vi "Field Types.vi"() -> (3 "Creatable Field Types":refnum<class "Type.lvclass">[](array[class]))   [LabVIEW 2020, in "Conditum-Tools.lvlib"]
uses:
  Conditum-Tools.lvlib
  Conditum-Clone/Columns/Type/Type.lvclass
  Conditum-Clone/Columns/Boolean/Boolean.lvclass
  C:/dev/lv20CE/lv-conditum-tools/Conditum-Clone/Columns/Type/Type.lvclass
  Conditum-Clone/Columns/Double/Double.lvclass
  Conditum-Clone/Columns/Integer/Integer.lvclass
  Conditum-Clone/Columns/String/String.lvclass
  Conditum-Clone/Columns/Text/Text.lvclass
  Conditum-Clone/Columns/Timestamp/Timestamp.lvclass
  Conditum-Clone/Columns/Relation/Relation.lvclass
  C:/dev/lv20CE/lv-conditum-tools/Conditum-Clone/Columns/Boolean/Boolean.lvclass
  C:/dev/lv20CE/lv-conditum-tools/Conditum-Clone/Columns/Double/Double.lvclass
  C:/dev/lv20CE/lv-conditum-tools/Conditum-Clone/Columns/Integer/Integer.lvclass
  C:/dev/lv20CE/lv-conditum-tools/Conditum-Clone/Columns/Timestamp/Timestamp.lvclass
  C:/dev/lv20CE/lv-conditum-tools/Conditum-Clone/Columns/Relation/Relation.lvclass
  C:/dev/lv20CE/lv-conditum-tools/Conditum-Clone/Columns/String/String.lvclass
  C:/dev/lv20CE/lv-conditum-tools/Conditum-Clone/Columns/Text/Text.lvclass
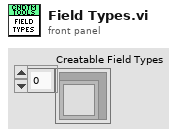
[diagram p1: front panel]
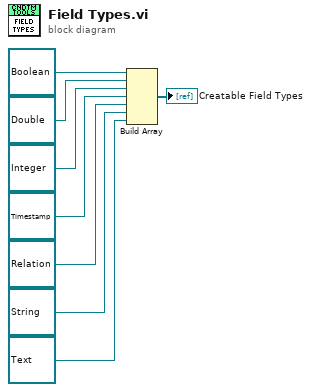
[diagram p0: block diagram]
diagram:
  n1 = Build Array(refnum<class "Boolean.lvclass"> refnum ("Conditum:Columns:Boolean.lvclass"), refnum<class "Double.lvclass"> refnum ("Conditum:Columns:Double.lvclass"), refnum<class "Integer.lvclass"> refnum ("Conditum:Columns:Integer.lvclass"), refnum<class "Timestamp.lvclass"> refnum ("Conditum:Columns:Timestamp.lvclass"), refnum<class "Relation.lvclass"> refnum ("Conditum:Columns:Relation.lvclass"), refnum<class "String.lvclass"> refnum ("Conditum:Columns:String.lvclass"), refnum<class "Text.lvclass"> refnum ("Conditum:Columns:Text.lvclass")) -> (→"Creatable Field Types":refnum<class "Type.lvclass">[])
